vi "Draw Frame.vi"(7 "Bounds":T1={"left"=0, "top"=0, "right"=150, "bottom"=100}, 11 "Picture In":picture) -> (3 "Picture":picture)   [LabVIEW 2022 SP3, in "FlexBlocks Support.lvlib"]
uses:
  FlexBlocks Support.lvlib
  Corner.ctl
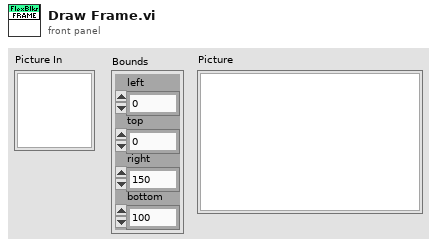
[diagram p1: front panel]
types:
  T1 = cluster{"left":i16, "top":i16, "right":i16, "bottom":i16}
  T2 = typedef "FlexBlocks Support.lvlib/Corner.ctl" = enum16{"TL", "TR", "BL", "BR"}
  T3 = typedef "imagedata.ctl" = cluster{"image type":i32, "image depth":i32, "image":u8[], "mask":u8[], "colors":u32[], "Rectangle":cluster{"left":i16, "top":i16, "right":i16, "bottom":i16}}
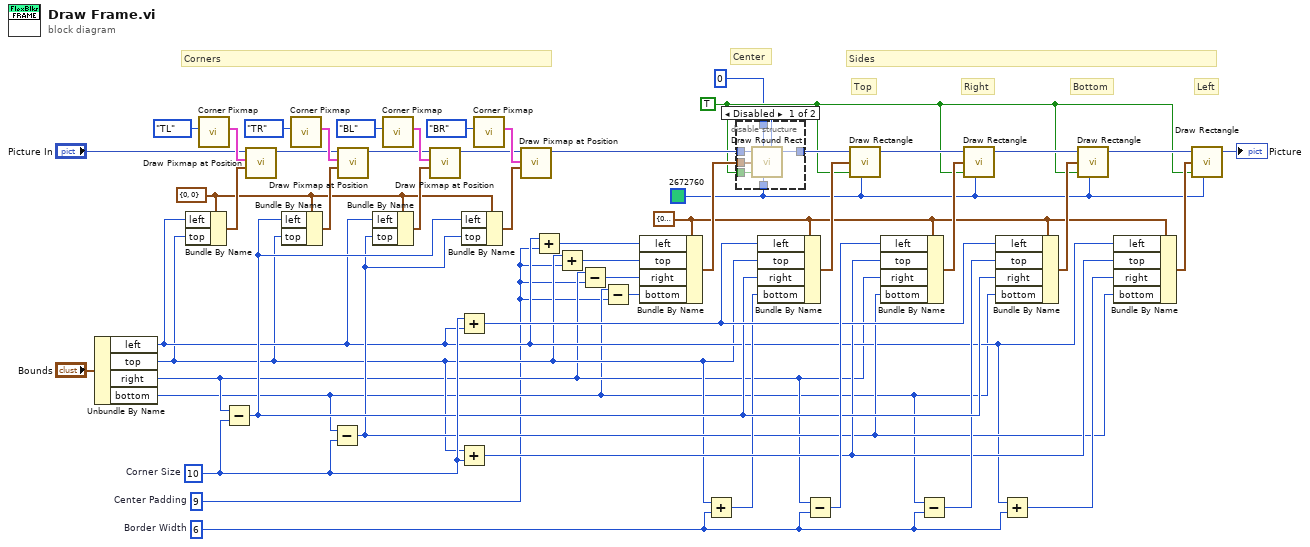
[diagram p0: block diagram]
diagram:
  w2 = i16 9  # Center Padding
  w13 = i16 6  # Border Width
  w20 = u32 2672760 ("color(black)")
  w11 = TRUE ("fill?(F)")
  w23 = T1 {"left"=0, "top"=0, "right"=0, "bottom"=0} ("rect")
  w33 = i16 10  # Corner Size
  w35 = cluster{"left":i16, "top":i16} {"left"=0, "top"=0} ("Position")
  # "Corners"
  # "Sides"
  # "Center"
  # "Left"
  # "Bottom"
  # "Right"
  # "Top"
  n1 = Unbundle By Name("Bounds") -> ("left"=w10:i16, "top"=w5:i16, "right"=w4:i16, "bottom"=w3:i16)
  n2 = Bundle By Name(cluster=w35, "left"=w10, "top"=w5) -> (w38:cluster{"left":i16, "top":i16})
  n3 = call "Corner Pixmap.vi"("Corner"=Corner."TL") -> ("Corner Pixmap"=w51:T3)  [unwired: 10 in]
  n4 = Subtract(x=w4, y=w33) -> (x-y=w18:i16)
  n5 = call "Draw Pixmap at Position.vi"("Position"=w38, "Pixmap"=w51, "2D Picture In"="Picture In") -> ("2D Picture"=w44:picture)  [unwired: 8 in]
  n6 = Bundle By Name(cluster=w35, "left"=w18, "top"=w5) -> (w37:cluster{"left":i16, "top":i16})
  n7 = call "Corner Pixmap.vi"("Corner"=Corner."TR") -> ("Corner Pixmap"=w50:T3)  [unwired: 10 in]
  n8 = Subtract(x=w3, y=w33) -> (x-y=w12:i16)
  n9 = call "Draw Pixmap at Position.vi"("Position"=w37, "Pixmap"=w50, "2D Picture In"=w44) -> ("2D Picture"=w43:picture)  [unwired: 8 in]
  n10 = Bundle By Name(cluster=w35, "left"=w10, "top"=w12) -> (w36:cluster{"left":i16, "top":i16})
  n11 = call "Corner Pixmap.vi"("Corner"=Corner."BL") -> ("Corner Pixmap"=w46:T3)  [unwired: 10 in]
  n12 = call "Draw Pixmap at Position.vi"("Position"=w36, "Pixmap"=w46, "2D Picture In"=w43) -> ("2D Picture"=w42:picture)  [unwired: 8 in]
  n13 = Add(x=w33, y=w10) -> (x+y=w19:i16)
  n14 = Add(x=w5, y=w33) -> (x+y=w16:i16)
  n15 = Bundle By Name(cluster=w35, "left"=w18, "top"=w12) -> (w34:cluster{"left":i16, "top":i16})
  n16 = call "Corner Pixmap.vi"("Corner"=Corner."BR") -> ("Corner Pixmap"=w45:T3)  [unwired: 10 in]
  n17 = call "Draw Pixmap at Position.vi"("Position"=w34, "Pixmap"=w45, "2D Picture In"=w42) -> ("2D Picture"=w41:picture)  [unwired: 8 in]
  n18 = Add(x=w10, y=w2) -> (x+y=w9:i16)
  n19 = Add(x=w5, y=w2) -> (x+y=w8:i16)
  n20 = Subtract(x=w4, y=w2) -> (x-y=w7:i16)
  n21 = Subtract(x=w3, y=w2) -> (x-y=w6:i16)
  n22 = Bundle By Name(cluster=w23, "left"=w9, "top"=w8, "right"=w7, "bottom"=w6) -> (w32:T1)
  n23 = Add(x=w5, y=w13) -> (x+y=w14:i16)
  n24 = disable-structure shown="Disabled" {
    disable-tunnel: w41 -> [w58 w59]
    disable-tunnel: w32 -> [w57 _]
    disable-tunnel: [w56 w59] -> w31
    disable-tunnel: w20 -> [w55 _]
    disable-tunnel: w11 -> [w54 _]
    disable-tunnel: i16 0 ("oval width") -> [w53 _]
    frame Disabled {
      n25 = call <vilib>:"Draw Round Rect.vi"("picture"=w58, "oval width"=w53, "rect"=w57, "fill?(F)"=w54, "color(black)"=w55, "oval height"=w53) -> ("new picture"=w56:picture)  [unwired: 3 in]
    }
    frame Enabled {
    }
  }
  n26 = Bundle By Name(cluster=w23, "left"=w19, "top"=w5, "right"=w18, "bottom"=w14) -> (w26:T1)
  n27 = Subtract(x=w4, y=w13) -> (x-y=w21:i16)
  n28 = call <vilib>:"Draw Rectangle.vi"("picture"=w31, "rect"=w26, "fill?(F)"=w11, "color(black)"=w20) -> ("new picture"=w30:picture)  [unwired: 5 in]
  n29 = Bundle By Name(cluster=w23, "left"=w21, "top"=w16, "right"=w4, "bottom"=w12) -> (w25:T1)
  n30 = Subtract(x=w3, y=w13) -> (x-y=w17:i16)
  n31 = call <vilib>:"Draw Rectangle.vi"("picture"=w30, "rect"=w25, "fill?(F)"=w11, "color(black)"=w20) -> ("new picture"=w29:picture)  [unwired: 5 in]
  n32 = Bundle By Name(cluster=w23, "left"=w19, "top"=w17, "right"=w18, "bottom"=w3) -> (w24:T1)
  n33 = Add(x=w10, y=w13) -> (x+y=w15:i16)
  n34 = call <vilib>:"Draw Rectangle.vi"("picture"=w29, "rect"=w24, "fill?(F)"=w11, "color(black)"=w20) -> ("new picture"=w28:picture)  [unwired: 5 in]
  n35 = Bundle By Name(cluster=w23, "left"=w10, "top"=w16, "right"=w15, "bottom"=w12) -> (w22:T1)
  n36 = call <vilib>:"Draw Rectangle.vi"("picture"=w28, "rect"=w22, "fill?(F)"=w11, "color(black)"=w20) -> ("new picture"=→"Picture":picture)  [unwired: 5 in]
